vi "XML Script - Append Terminal Name.vi"   [LabVIEW 2017]
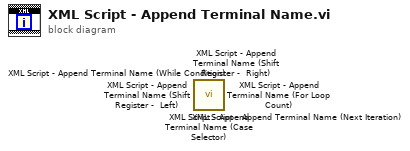
[diagram p0: block diagram]
diagram:
  n1 = call <vilib>:"XML Script - Append Terminal Name (Case Selector).vi"() -> ()  [unwired: 1 in, 1 out]
  n2 = call <vilib>:"XML Script - Append Terminal Name (Shift Register -  Right).vi"() -> ()  [unwired: 1 in, 1 out]
  n3 = call <vilib>:"XML Script - Append Terminal Name (Shift Register -  Left).vi"() -> ()  [unwired: 1 in, 1 out]
  n4 = call <vilib>:"XML Script - Append Terminal Name (For Loop Count).vi"() -> ()  [unwired: 1 in, 1 out]
  n5 = call <vilib>:"XML Script - Append Terminal Name (While Condition).vi"() -> ()  [unwired: 1 in, 1 out]
  n6 = call <vilib>:"XML Script - Append Terminal Name (Next Iteration).vi"() -> ()  [unwired: 1 in, 1 out]
